vi "Cycle Read.vi"(4 "error in (no error)":errorcluster, 6 "Container State":T2, 7 "Display State In":T1={"cycle"=1.0, "timing vi"=refnum, "event"=refnum}) -> (0 "error out":errorcluster, 2 "Value":dbl=1.0, 3 "Display State Out":T1={"cycle"=1.0, "timing vi"=refnum, "event"=refnum})   [LabVIEW 2024, in "Twinkle Button.xctl"]
doc: "本VI是为《我和LabVIEW》一书编写的示例。\n关于本书的介绍请参考网页：\nhttp://ruanqizhen.spaces.live.com/blog/cns!5852D4F797C53FB6!4310.entry"
uses:
  Twinkle Button.xctl
  <vilib>/_xctls/Container State.ctl
  State.ctl
  <resource>/importtools/Common/Event/NISAST Event.lvclass
  <vilib>/_xctls/XControlSupport.lvlib
panel:
  # "Replace the Value Indicator below with an Indicator of desired type.\nDo not remove this Indicator or the others from the connector pane. \nDo not change the connector pane pattern.\nThe Value Indicator should always be the second terminal from top on the output side in the connector pane."
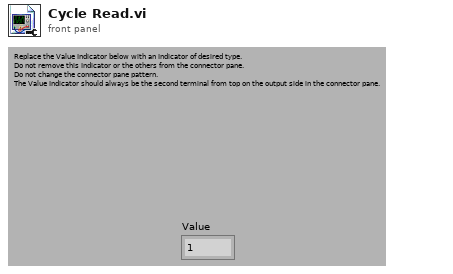
[diagram p1: front panel]
types:
  T1 = typedef "Twinkle Button.xctl/State.ctl" = cluster{"cycle":dbl, "timing vi":refnum<vi>, "event":refnum<class "NISAST Event.lvclass">}
  T2 = typedef "XControlSupport.lvlib/Container State.ctl" = cluster{"Indicator?":bool, "Run Mode?":bool, " Refnum":refnum<vi>}
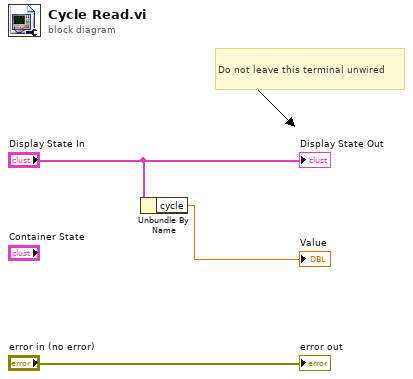
[diagram p0: block diagram]
diagram:
  # "Do not leave this terminal unwired"
  n1 = Unbundle By Name("Display State In") -> ("cycle"=→"Value":dbl)
  "error out" <- "error in (no error)"
  "Display State Out" <- "Display State In"
